vi "StopAllStageDll.vi"(8 "error in":errorcluster, 11 "DevRefIn":u32) -> (0 "error out":errorcluster, 2 "result string":string, 3 "DevRefOut":u32)   [LabVIEW 2020]
uses:
  gclib32.lvlib
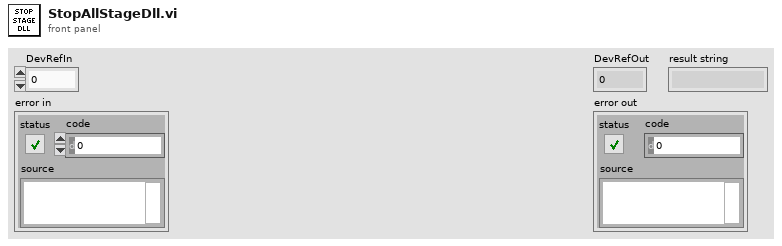
[diagram p1: front panel]
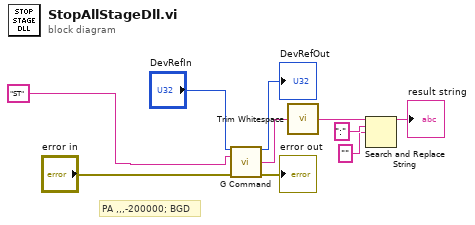
[diagram p0: block diagram]
diagram:
  # "PA ,,,-200000; BGD"
  n1 = call "G Command.vi"("g"="DevRefIn", "command"="ST" ("format string"), "error in (no error)"="error in") -> ("g out"=→"DevRefOut":u32, "buffer out"=w5:string, "error out"=→"error out":errorcluster)  [unwired: 10 in]
  n2 = call "Trim Whitespace.vi"("string"=w5) -> ("trimmed string"=w10:string)  [unwired: 1 in]
  n3 = Search and Replace String(input string=w10, search string=":", replace string="" ("replace string (\"\")")) -> (result string=→"result string":string)  [unwired: 5 in, 3 out]
